vi "通过CMD打开任意文件.vi"(11 "路径 2":path) -> ()   [LabVIEW 2018]
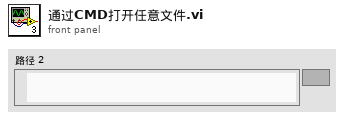
[diagram p1: front panel]
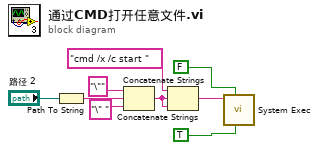
[diagram p0: block diagram]
diagram:
  n1 = Path To String(path="路径 2") -> (string=w6:string)
  n2 = Concatenate Strings("\"" ("Substring"), w6, "\" " ("Substring")) -> (w7:string)
  n3 = Concatenate Strings("cmd /x /c start ", w7, w7) -> (w3:string)
  n4 = call <vilib>:"System Exec.vi"("run minimized? (F)"=TRUE, "wait until completion? (T)"=FALSE ("Wait until done"), "command line"=w3) -> ()  [unwired: 3 in, 6 out]
